vi "Write Build Machine Feed Folderpath.vi"(8 "error in (no error)":errorcluster, 10 "Build Machine Feed Folderpath":path, 11 "NIPKG_LV in":refnum<class "NIPKG_LV.lvclass">) -> (0 "error out":errorcluster, 3 "NIPKG_LV out":refnum<class "NIPKG_LV.lvclass">)   [LabVIEW 2017, in "CL_G3_VIComponentBuilder.lvlib" / "NIPKG_LV.lvclass"]
uses:
  NIPKG_LV.lvclass
  NIPKG_LV.lvclass/NIPKG_LV.ctl
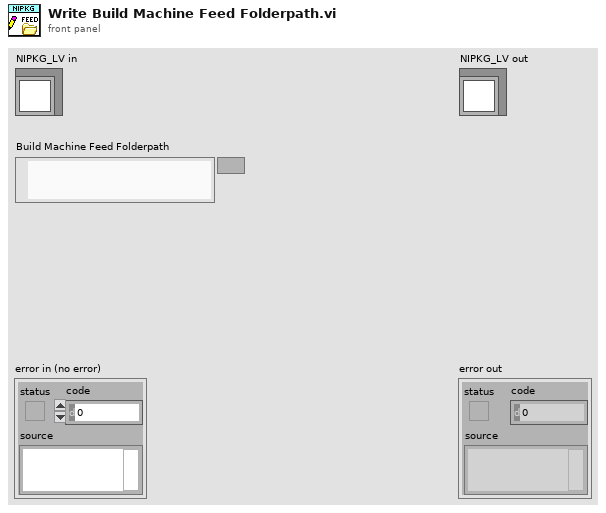
[diagram p1: front panel]
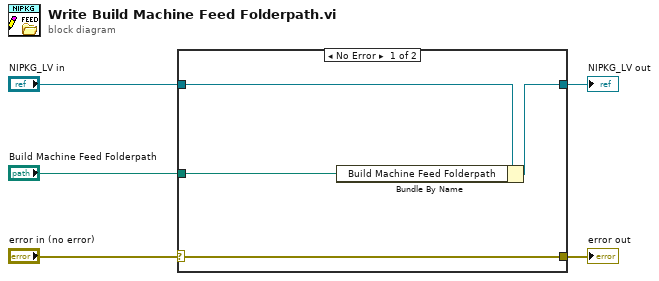
[diagram p0: block diagram]
diagram:
  n1 = case shown="No Error" "error in (no error)" {
    selector: "error in (no error)" -> [w9 w10]
    tunnel: [w9 w10] -> w4
    tunnel: [w7 w11] -> w2
    tunnel: "NIPKG_LV in" -> [w8 w11]
    tunnel: "Build Machine Feed Folderpath" -> [w6 _]
    frame No Error {
      n2 = Bundle By Name(cluster=w8, "Build Machine Feed Folderpath"=w6) -> (w7:refnum<class "NIPKG_LV.lvclass">)
    }
    frame Error {
    }
  }
  "error out" <- w4
  "NIPKG_LV out" <- w2
